vi "Launcher.vi"() -> ()   [LabVIEW 2018]
panel:
  out "error out 2":errorcluster
  out "Array":errorcluster[](array[cluster])
  out "error out":errorcluster
  in  "Feed Module 4":bool
  in  "Feed Module 3":bool
  in  "Feed Module 2":bool
  in  "Exit Button":bool
  in  "Feed Module 1":bool
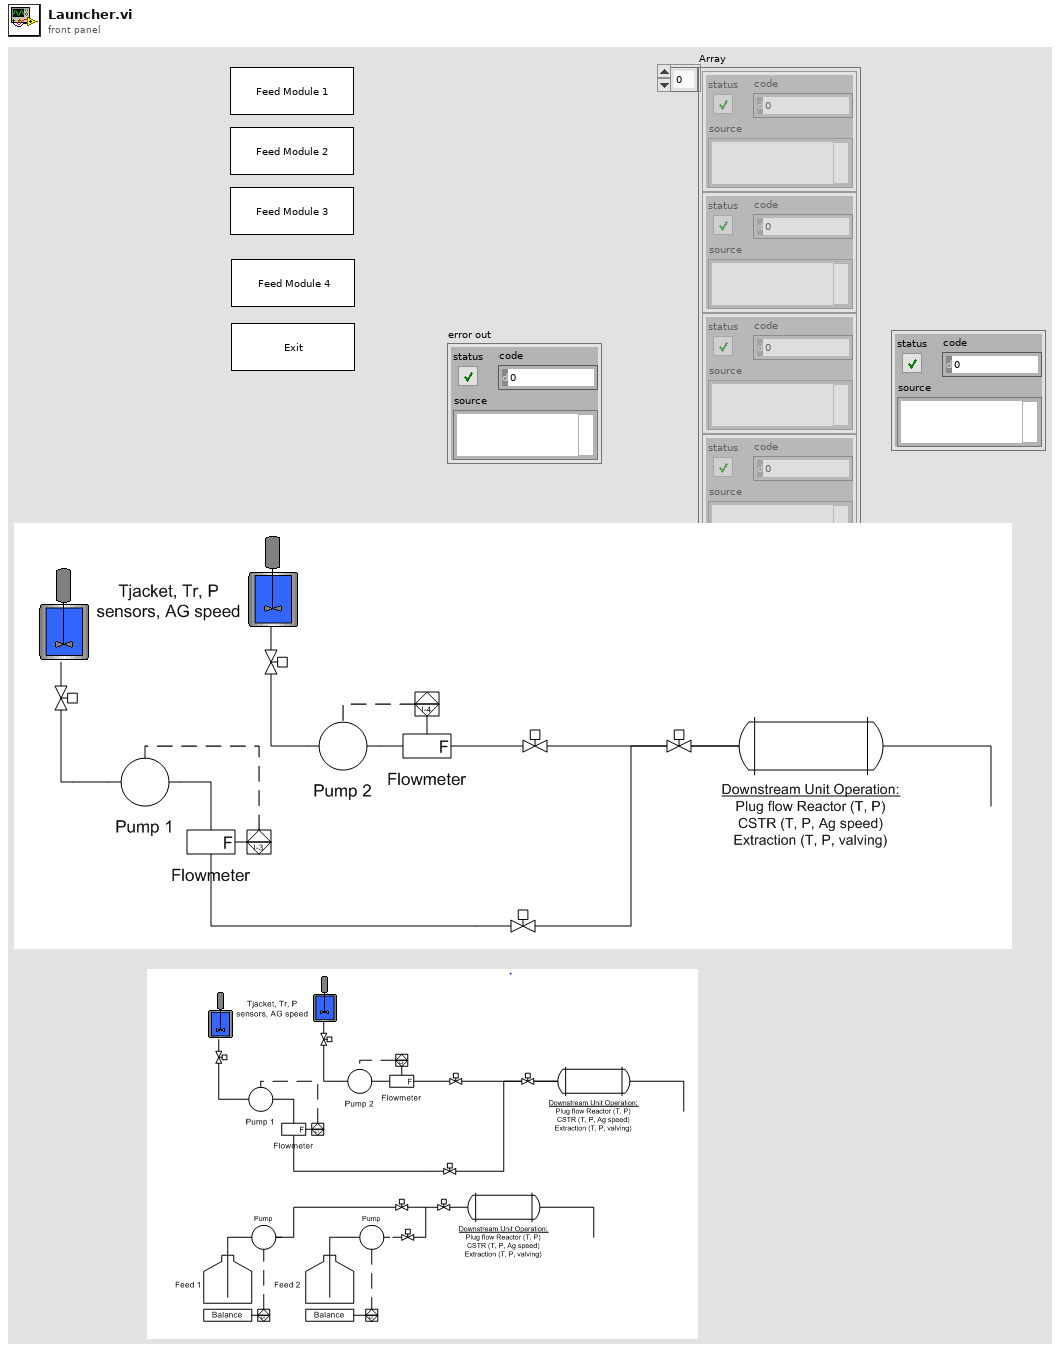
[diagram p1: front panel]
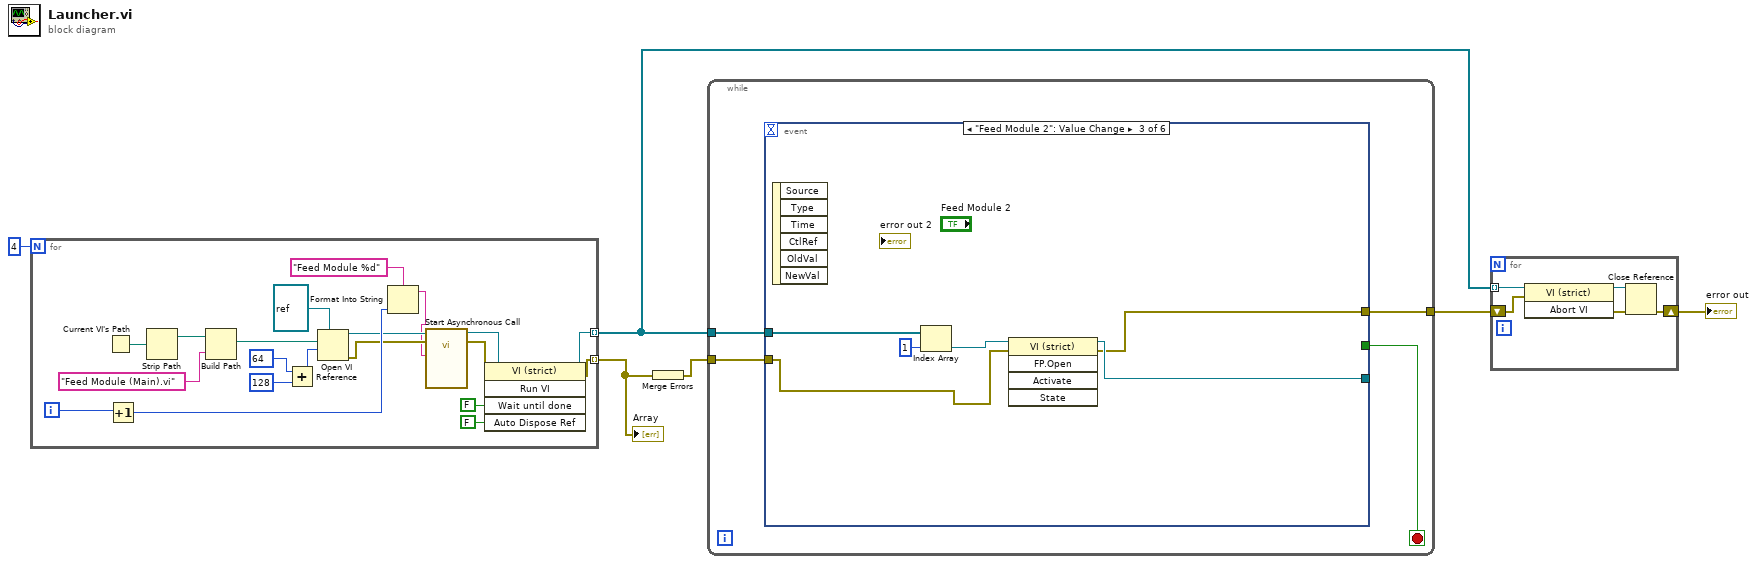
[diagram p0: block diagram]
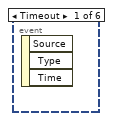
[diagram p2: hidden frame]
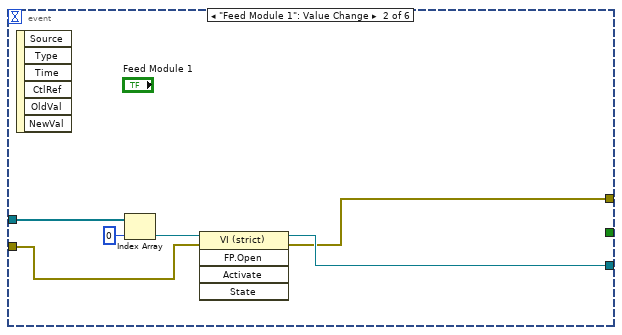
[diagram p3: hidden frame]
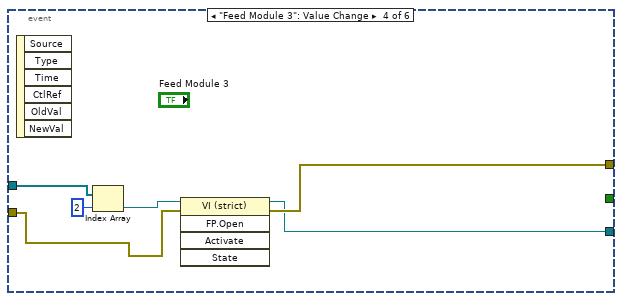
[diagram p4: hidden frame]
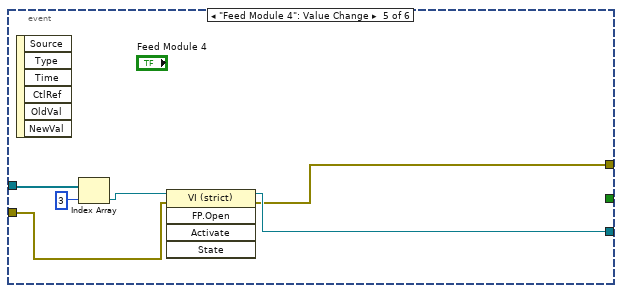
[diagram p5: hidden frame]
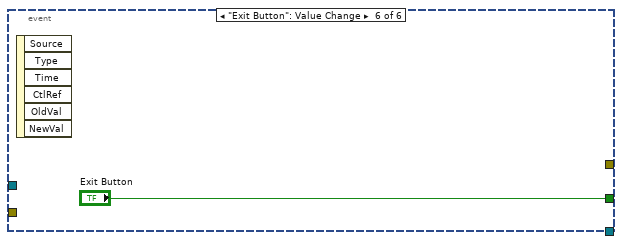
[diagram p6: hidden frame]
diagram:
  n1 = for {
    N: 4 -> [_]
    tunnel: [w9] -> w3 mode=indexing
    tunnel: [w11] -> w2 mode=indexing
    i -> [w17]
    n2 = Current VI's Path() -> (path=w23:path)
    n3 = Increment(x=w17) -> (x+1=w16:i32)
    n4 = Strip Path(path=w23) -> (stripped path=w24:path)  [unwired: 1 out]
    n5 = Build Path(base path=w24, name or relative path="Feed Module (Main).vi") -> (appended path=w25:path)
    n6 = Add(x=64 ("options"), y=128 ("options")) -> (x+y=w26:i32)
    n7 = Open VI Reference(type specifier VI Refnum (for type only)=refnum<vi> refnum, vi path=w25, options=w26) -> (vi reference=w15:refnum<vi>, error out=w14:errorcluster)  [unwired: 3 in]
    n8 = Format Into String(format string="Feed Module %d", w16) -> (resulting string=w13:string)  [unwired: 2 in, 1 out]
    n9 = call-by-ref "Start Asynchronous Call"(reference=w15, error in=w14, "Process Name"=w13) -> (reference out=w10:refnum<vi>, error out=w12:errorcluster)  [unwired: 11 in]
    n10 = invoke class="VI (strict)" method="Run VI"(reference=w10, error in=w12, "Wait until done"=FALSE ("Wait Until Done"), "Auto Dispose Ref"=FALSE ("Auto Dispose Reference")) -> (reference out=w9:refnum<vi>, error out=w11:errorcluster)  [unwired: 1 in, 3 out]
  }
  "Array" <- w2
  n11 = Merge Errors(w2) -> (w1:errorcluster)
  n12 = while {
    tunnel: w3 -> [w29]
    tunnel: w1 -> [w28]
    tunnel: [w27] -> w4
    stop <- w30 stop-if-true
    n13 = event shown="[2] \"Feed Module 2\": Value Change" {
      selector: _ -> [_ _ _ _ _ _]
      dyn-events: _ -> [_ _ _ _ _ _]
      timeout: _ -> [_ _ _ _ _ _]
      tunnel: [_ _ _ _ _ "Exit Button"] -> w30
      tunnel: [_ w33 w38 w45 w50 _] -> w27
      tunnel: w29 -> [_ w35 w40 w46 w54 _]
      tunnel: w28 -> [_ w31 w37 w43 w49 _]
      tunnel: [_ w34 w39 w44 w51 _] -> _
      event Timeout {
        n14 = event-data() -> ()  [unwired: 1 in, 3 out]
      }
      event "Feed Module 1": Value Change {
        n15 = event-data() -> ()  [unwired: 1 in, 6 out]
        n16 = Index Array(array=w35, index=0) -> (element=w32:refnum<vi>)
        n17 = invoke class="VI (strict)" method="FP.Open"(reference=w32, error in=w31) -> (reference out=w34:refnum<vi>, error out=w33:errorcluster)  [unwired: 3 in, 3 out]
      }
      event "Feed Module 2": Value Change {
        n18 = event-data() -> ()  [unwired: 1 in, 6 out]
        n19 = Index Array(array=w40, index=1) -> (element=w41:refnum<vi>)
        n20 = invoke class="VI (strict)" method="FP.Open"(reference=w41, error in=w37) -> (reference out=w39:refnum<vi>, error out=w38:errorcluster)  [unwired: 3 in, 3 out]
      }
      event "Feed Module 3": Value Change {
        n21 = event-data() -> ()  [unwired: 1 in, 6 out]
        n22 = Index Array(array=w46, index=2) -> (element=w47:refnum<vi>)
        n23 = invoke class="VI (strict)" method="FP.Open"(reference=w47, error in=w43) -> (reference out=w44:refnum<vi>, error out=w45:errorcluster)  [unwired: 3 in, 3 out]
      }
      event "Feed Module 4": Value Change {
        n24 = event-data() -> ()  [unwired: 1 in, 6 out]
        n25 = Index Array(array=w54, index=3) -> (element=w52:refnum<vi>)
        n26 = invoke class="VI (strict)" method="FP.Open"(reference=w52, error in=w49) -> (reference out=w51:refnum<vi>, error out=w50:errorcluster)  [unwired: 3 in, 3 out]
      }
      event "Exit Button": Value Change {
        n27 = event-data() -> ()  [unwired: 1 in, 6 out]
      }
    }
  }
  n28 = for {
    shift-right: [w60] -> w5
    shift-left: w4 -> [w59]
    tunnel: w3 -> [w56] mode=indexing
    n29 = invoke class="VI (strict)" method="Abort VI"(reference=w56, error in=w59) -> (reference out=w58:refnum<vi>, error out=w57:errorcluster)  [unwired: 1 in, 1 out]
    n30 = Close Reference(reference=w58, error in (no error)=w57) -> (error out=w60:errorcluster)
  }
  "error out" <- w5
